vi "Remove Comment lines from 2D array of strings.vi"(1 "Array in":string[][](array[string])) -> (0 "Array out":string[][](array[string]))   [LabVIEW 2013]
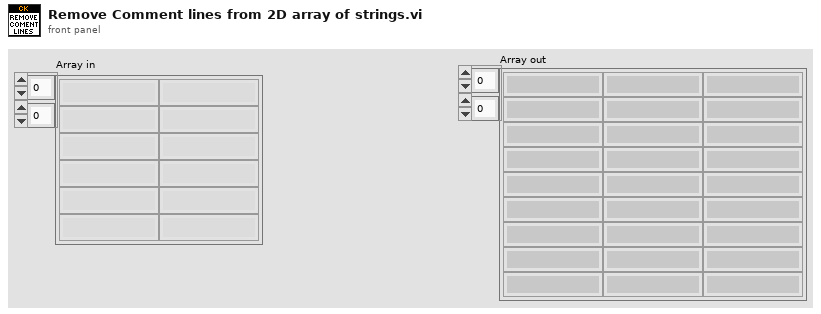
[diagram p1: front panel]
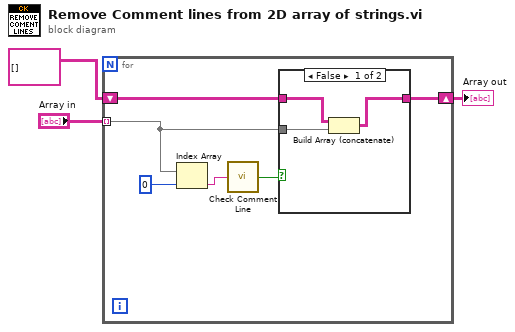
[diagram p0: block diagram]
diagram:
  n1 = for {
    tunnel: "Array in" -> [w7] mode=indexing
    shift-right: [w5] -> w2
    shift-left: string[][] [] -> [w6]
    n2 = Index Array(array=w7, index=0) -> (element=w8:string)
    n3 = call "Check Comment Line.vi"("String"=w8) -> ("Starts with #?"=w4:bool)
    n4 = case shown="False" w4 {
      tunnel: w7 -> [w12 _]
      tunnel: w6 -> [w11 w13]
      tunnel: [w10 w13] -> w5
      frame False {
        n5 = Build Array (concatenate)(w11, w12) -> (w10:string[][])
      }
      frame True {
      }
    }
  }
  "Array out" <- w2
